vi "WPI_Camera Connection Responder.vi"(11 "connection ID":refnum<k5>) -> ()   [LabVIEW 2017]
uses:
  <vilib>/Rock Robotics/SystemInterfaces/NetworkCommunication/NetComm_UsageReport_ResourceType.ctl
  <vilib>/Rock Robotics/WPI/Camera/WPI_CameraImageSize.ctl
  <vilib>/Utility/error.llb/Error Cluster From Error Code.vi
  <vilib>/ErrorRing/Error Ring.xnode
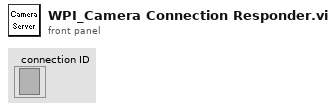
[diagram p1: front panel]
types:
  T1 = typedef "NetComm_UsageReport_ResourceType.ctl" = enum8{"Controller", "Module", "Language", "CANPlugin", "Accelerometer", "ADXL345", "AnalogChannel", "AnalogTrigger", "AnalogTriggerOutput", "CANJaguar", "Compressor", "Counter", "Dashboard", "DigitalInput", "DigitalOutput", "DriverStationCIO", "DriverStationEIO", "DriverStationLCD", "Encoder", "GearTooth", "Gyro", "I2C", "Framework", "Jaguar", "Joystick", "Kinect", "KinectStick", "PIDController", "Preferences", "PWM", "Relay", "RobotDrive", "SerialPort", "Servo", "Solenoid", "SPI", "Task", "Ultrasonic", "Victor", "Button", "Command", "AxisCamera", "PCVideoServer", "SmartDashboard", "Talon", "HiTechnicColorSensor", "HiTechnicAccel", "HiTechnicCompass", "SRF08", "AnalogOutput", "Victor SP", "Talon SRX", "CAN Talon SRX", "ADXL362 Accel", "ADXRS450 Gyro", "Rev SPARK", "Mindsensors SD540", "Digital Filter", "ADIS16448", "PDP", "PCM", "PigeonIMU", "Nidec Brushless", "CTRE CANifier", "CTRE Future 0", "CTRE Future 1", "CTRE Future 2", "CTRE Future 3", "CTRE Future 4", "CTRE Future 5", "CTRE Future 6"}
  T2 = cluster{"Camera Name":string, "Size":string, "Frame Rate":i32, "Compression":i32}
  T3 = enum16{"Standard", "Buffered", "CRLF", "Immediate"}
  T4 = typedef "WPI_CameraImageSize.ctl" = enum16{"640x480", "320x240", "160x120", "Custom"}
  T5 = enum16{"Update Mode", "Get Image", "Get Image Data"}
  T6 = typedef "Image Type" = u32
  T7 = typedef "WPI_CameraDevRef.ctl" = cluster{"Camera Address":string, "CameraStatus":errorcluster}
  T8 = typedef "IMAQ Image.ctl" = refnum<image>
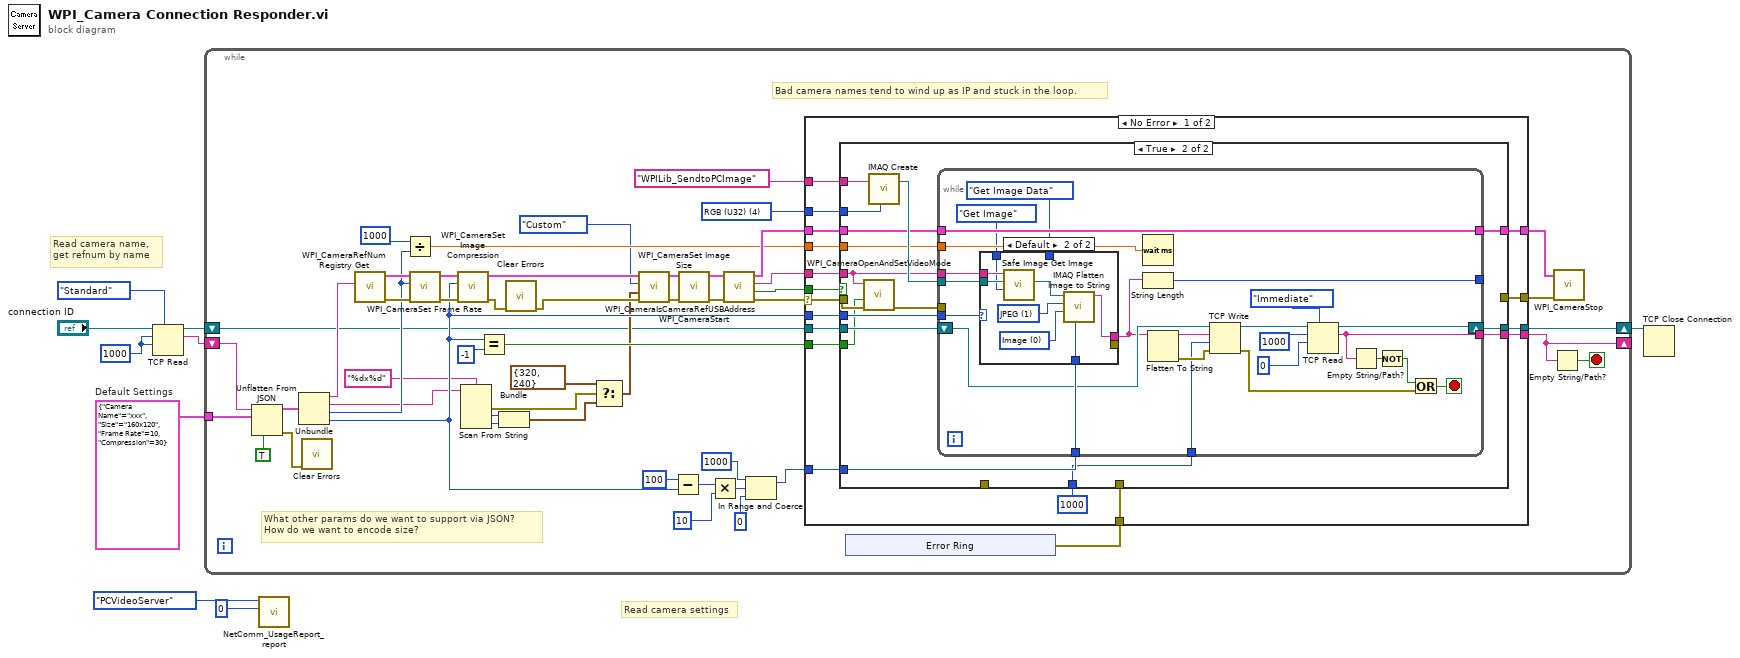
[diagram p0: block diagram]
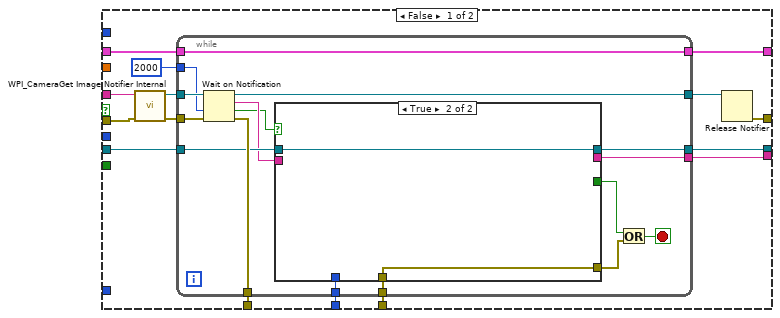
[diagram p2: hidden frame]
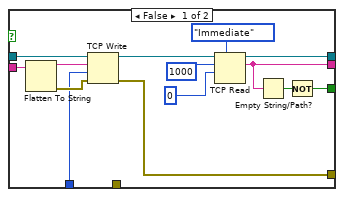
[diagram p3: hidden frame]
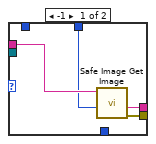
[diagram p4: hidden frame]
diagram:
  w5 = T2 {"Camera Name"="xxx", "Size"="160x120", "Frame Rate"=10, "Compression"=30}  # Default Settings
  w4 = 1000
  # "Read camera settings"
  # "Read camera name,\nget refnum by name"
  n1 = TCP Read(connection ID="connection ID", bytes to read=w4, 7:T3."Standard" ("mode (standard)"), 9:w4) -> (connection ID out=w6:refnum<k5>, data out=w3:string)  [unwired: 1 in, 1 out]
  n2 = while {
    tunnel: w5 -> [w33]
    shift-right: [w61] -> w9
    shift-left: w6 -> [w12]
    shift-right: [w11] -> _
    shift-left: w3 -> [w13]
    stop <- w10 stop-if-true
    w57 = T6 4 items=["Grayscale (U8)", "Grayscale (I16)", "Grayscale (SGL)", "Complex (CSG)", "RGB (U32)", "HSL (U32)", "RGB (U64)", "Grayscale (U16)"] ("Image Type")
    # "Bad camera names tend to wind up as IP and stuck in the loop."
    # "What other params do we want to support via JSON?\nHow do we want to encode size?"
    n3 = Unflatten From JSON(JSON string=w13, type and defaults=w33, default null elements? (F)=TRUE) -> (value=w31:T2, error out=w32:errorcluster)  [unwired: 4 in]
    n4 = Unbundle(w31) -> ("Camera Name"=w29:string, "Size"=w24:string, "Frame Rate"=w25:i32, "Compression"=w26:i32)
    n5 = call <vilib>:"Clear Errors.vi"("error in (no error)"=w32) -> ()  [unwired: 5 in, 2 out]
    n6 = call <vilib>:"WPI_CameraRefNum Registry Get.vi"("refnum name"=w29) -> ("error out"=w27:errorcluster, "CameraDevRef"=w28:T7)  [unwired: 9 in]
    n7 = Divide(x=u16 1000 ("port"), y=w25) -> (x/y=w45:dbl)
    n8 = call <vilib>:"WPI_CameraSet Frame Rate.vi"("error in (no error)"=w27, "Frame Rate (fps)"=w25, "CameraDevRef"=w28) -> ("error out"=w48:errorcluster, "CameraDevRef Out"=w51:T7)  [unwired: 7 in]
    n9 = call <vilib>:"WPI_CameraSet Image Compression.vi"("error in (no error)"=w48, "Compression"=w26, "CameraDevRef"=w51) -> ("error out"=w35:errorcluster, "CameraDevRef Out"=w50:T7)  [unwired: 7 in]
    n10 = Scan From String(format string="%dx%d", input string=w24) -> (error out=w19:errorcluster, output 1=w22:i32, output 2=w21:i32)  [unwired: 4 in, 2 out]
    n11 = Equal?(x=w26, y=-1) -> (x = y?=w36:bool)
    n12 = Bundle(w22, w21) -> (w18:cluster{i32, i32})  [unwired: 1 in]
    n13 = call <vilib>:"Clear Errors.vi"("error in (no error)"=w35) -> ("error out"=w34:errorcluster)  [unwired: 5 in, 1 out]
    n14 = Select(t=cluster{i32, i32} {320, 240} ("s? t:f"), s=w19, f=w18) -> (s? t:f=w17:cluster{i32, i32})
    n15 = call <vilib>:"WPI_CameraSet Image Size.vi"("error in (no error)"=w34, "Size W,H (pix)"=w17, "Image Size"=WPI_CameraImageSize."Custom", "CameraDevRef"=w50) -> ("error out"=w47:errorcluster, "CameraDevRef Out"=w49:T7)  [unwired: 6 in]
    n16 = Subtract(x=100, y=w26) -> (x-y=w40:i32)
    n17 = call <vilib>:"WPI_CameraStart.vi"("error in (no error)"=w47, "CameraDevRef"=w49) -> ("error out"=w54:errorcluster, "CameraDevRef"=w53:T7)  [unwired: 8 out]
    n18 = Multiply(x=w40, y=10) -> (x*y=w42:i32)
    n19 = call <vilib>:"WPI_CameraIsCameraRefUSBAddress.vi"("error in (no error)"=w54, "CameraDevRef"=w53) -> ("error out"=w15:errorcluster, "USB?"=w55:bool, "Camera Address Out"=w56:string, "CameraDevRef out"=w52:T7)  [unwired: 6 in]
    n20 = In Range and Coerce(upper limit=1000, x=w42, lower limit=0) -> (coerced(x)=w38:i32)  [unwired: 1 out]
    n21 = xnode "Error Ring"() -> ("error out"=w14:errorcluster)
    n22 = case shown="No Error" w15 {
      selector: w15 -> [w68 w183]
      tunnel: [w82 w182] -> w61
      tunnel: [w81 w184] -> w60
      tunnel: [w80 w183] -> w59
      tunnel: "WPILib_SendtoPCImage" -> [w79 _]
      tunnel: w57 -> [w78 _]
      tunnel: w56 -> [w77 _]
      tunnel: w55 -> [w76 _]
      tunnel: w52 -> [w75 w184]
      tunnel: w45 -> [w74 _]
      tunnel: w38 -> [w73 _]
      tunnel: w36 -> [w72 _]
      tunnel: w12 -> [w71 w182]
      tunnel: w26 -> [w70 _]
      tunnel: w14 -> [w67 _]
      tunnel: [w66 _] -> w11
      frame No Error {
        n23 = case shown="True" w76 {
          tunnel: w71 -> [w97 w145]
          tunnel: [w96 _] -> _
          tunnel: [w95 w144] -> w82
          tunnel: w68 -> [w94 w135]
          tunnel: w77 -> [w92 w134]
          tunnel: [w91 w139] -> w81
          tunnel: w75 -> [w90 w140]
          tunnel: [w88 _] -> w80
          tunnel: w79 -> [_ w142]
          tunnel: w78 -> [_ w141]
          tunnel: w73 -> [_ w138]
          tunnel: w74 -> [_ w137]
          tunnel: w70 -> [_ w136]
          tunnel: w72 -> [_ w132]
          tunnel: 1000 ("timeout ms (25000)") -> [w86 w131]
          tunnel: w67 -> [w85 _]
          tunnel: [w84 w130] -> w66
          frame False {
            n24 = call <vilib>:"WPI_CameraGet Image Notifier Internal.vi"("error in (no error)"=w94, "Camera Address"=w92) -> ("error out"=w93:errorcluster, "Image Notifier"=w89:refnum<notifier>)  [unwired: 8 out]
            n25 = while {
              tunnel: w93 -> [w112]
              tunnel: w97 -> [w107]
              tunnel: [w110] -> w96
              tunnel: [w106] -> w95
              tunnel: [w113] -> w91
              tunnel: w90 -> [w113]
              tunnel: w89 -> [w111]
              tunnel: [w109] -> w87
              tunnel: w86 -> [w108]
              tunnel: w85 -> [w103]
              tunnel: [w102] -> w84
              tunnel: 2000 ("Timeout in ms (-1)") -> [w100]
              stop <- w98 stop-if-true
              n26 = Wait on Notification(notifier=w111, timeout in ms (-1)=w100, error in (no error)=w112) -> (notifier out=w109:refnum<notifier>, notification=w105:string, timed out?=w104:bool, error out=w110:errorcluster)  [unwired: 1 out]
              n27 = case shown="True" w104 {
                tunnel: [w125 w128] -> w99
                tunnel: w108 -> [w124 _]
                tunnel: w107 -> [w123 w129]
                tunnel: [w117 w129] -> w106
                tunnel: w105 -> [w122 _]
                tunnel: w103 -> [_ w128]
                tunnel: [w116 _] -> w102
                tunnel: [w114 _] -> w101
                frame False {
                  n28 = Flatten To String(anything=w122) -> (data string=w127:string, error out=w126:errorcluster)  [unwired: 1 in, 3 out]
                  n29 = TCP Write(connection ID=w123, data in=w127, error in (no error)=w126, 9:w124) -> (connection ID out=w118:refnum<k5>, error out=w125:errorcluster)  [unwired: 1 out]
                  n30 = TCP Read(connection ID=w118, bytes to read=1000, 7:T3."Immediate" ("mode (standard)"), 9:0) -> (connection ID out=w117:refnum<k5>, data out=w116:string)  [unwired: 1 in, 1 out]
                  n31 = Empty String/Path?(string/path=w116) -> (empty?=w115:bool)
                  n32 = Not(x=w115) -> (.not. x?=w114:bool)
                }
                frame True {
                }
              }
              n33 = Or(x=w101, y=w99) -> (x .or. y?=w98:bool)
            }
            n34 = Release Notifier(notifier=w87) -> (error out=w88:errorcluster)  [unwired: 1 in, 3 out]
          }
          frame True {
            n35 = call <vilib>:"WPI_CameraOpenAndSetVideoMode.vi"("error in (no error)"=w135, "USB JPEG"=w132, "Camera Address"=w134) -> ("error out"=w133:errorcluster)  [unwired: 8 in]
            n36 = call "IMAQ Create"("Image Name"=w142, "Image Type"=w141) -> ("New Image"=w143:T8)  [unwired: 3 in, 1 out]
            n37 = while {
              tunnel: w134 -> [w169]
              shift-right: [w155] -> w144
              shift-left: w145 -> [w159]
              tunnel: w143 -> [w168]
              tunnel: [w167] -> w139
              tunnel: w140 -> [w167]
              tunnel: w138 -> [w166]
              tunnel: w137 -> [w165]
              tunnel: w136 -> [w164]
              tunnel: w133 -> [_]
              tunnel: w131 -> [w157]
              tunnel: [w154] -> w130
              tunnel: [w150] -> _
              stop <- w147 stop-if-true
              n38 = case shown="Default" w164 {
                tunnel: [w172 w181] -> w158
                tunnel: w169 -> [w173 w177]
                tunnel: w168 -> [_ w176]
                tunnel: w166 -> [_ w178]
                tunnel: [w171 _] -> _
                tunnel: T5."Get Image Data" ("Operation") -> [w170 _]
                tunnel: T5."Get Image" ("Operation") -> [_ w174]
                frame -1 {
                  n39 = call <vilib>:"Safe Image Get Image.vi"("Operation"=w170, "Session In"=w173) -> ("error out"=w171:errorcluster, "Image Data String"=w172:string)  [unwired: 6 in, 2 out]
                }
                frame Default {
                  w179 = 0 items=["Image", "Image and Vision Info", "Reference to Image"] ("Type of Flatten (Image and Vision Info)")
                  w180 = 1 items=["None", "JPEG", "PACKED BINARY"] ("Compression (None)")
                  n40 = call <vilib>:"Safe Image Get Image.vi"("Operation"=w174, "Image In"=w176, "Session In"=w177) -> ("Image Out"=w175:T8)  [unwired: 5 in, 3 out]
                  n41 = call "IMAQ Flatten Image to String"("Quality (750)"=w178, "Type of Flatten (Image and Vision Info)"=w179, "Compression (None)"=w180, "Image"=w175) -> ("Data String"=w181:string)  [unwired: 6 in, 1 out]
                }
              }
              n42 = Wait (ms)(milliseconds to wait=w165) -> ()  [unwired: 1 out]
              n43 = String Length(string=w158) -> (length=w150:i32)
              n44 = Flatten To String(anything=w158) -> (data string=w161:string, error out=w160:errorcluster)  [unwired: 1 in, 3 out]
              n45 = TCP Write(connection ID=w159, data in=w161, error in (no error)=w160, 9:w157) -> (connection ID out=w156:refnum<k5>, error out=w149:errorcluster)  [unwired: 1 out]
              n46 = TCP Read(connection ID=w156, bytes to read=1000, 7:T3."Immediate" ("mode (standard)"), 9:0) -> (connection ID out=w155:refnum<k5>, data out=w154:string)  [unwired: 1 in, 1 out]
              n47 = Empty String/Path?(string/path=w154) -> (empty?=w148:bool)
              n48 = Not(x=w148) -> (.not. x?=w146:bool)
              n49 = Or(x=w146, y=w149) -> (x .or. y?=w147:bool)
            }
          }
        }
      }
      frame Error {
      }
    }
    n50 = Empty String/Path?(string/path=w11) -> (empty?=w10:bool)
    n51 = call <vilib>:"WPI_CameraStop.vi"("error in (no error)"=w59, "CameraDevRef"=w60) -> ()  [unwired: 10 out]
  }
  n52 = call <vilib>:"NetComm_UsageReport_report.vi"("Instance Number"=u8 0, "Resource Type"=NetComm_UsageReport_ResourceType."PCVideoServer") -> ()  [unwired: 10 in]
  n53 = TCP Close Connection(connection ID=w9) -> ()  [unwired: 1 in, 3 out]
